vi "Pressure-Main-temp.vi"(8 "error in":errorcluster) -> (0 "error out":errorcluster)   [LabVIEW 2016]
doc: "Use this template to build a simple state machine design pattern. Each state executes code and determines which state to transition to."
uses:
  Controls/Pressure-Data.ctl
  Sensor-Class/Pressure-Transducer_class/Pressure-Transducer.lvclass
  Controls/Pressure-State.ctl
  Pressure Module.lvlib
panel:
  out "output array":u16[](array[numeric])
  out "Pressure":dbl[](array[numeric])
  out "Pressure 2":bool
  out "Status":string
  in  "Read Pressure":bool
  in  "Exit":bool
  # "P1"
  # "Flow 1"
  # "mA    Flow meter"
  # "Flow 2"
  # "mA  Flow meter"
  # "Top"
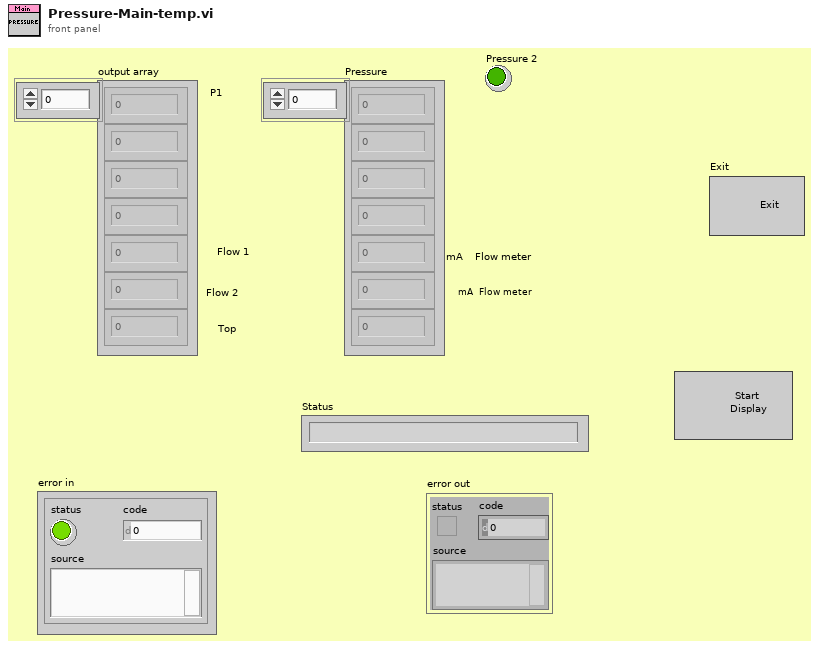
[diagram p1: front panel]
types:
  T1 = typedef "Pressure-State.ctl" = enum16{"Initialize", "Wait for Event", "Data: Pressure", "Data: Pressure-Sym", "Data: Display", "Data: Close", "Error", "Exit"}
  T2 = typedef "Pressure-Data.ctl" = cluster{"?":bool, "Status":string, "Pressure":dbl[], "Modbus-Instr":refnum<class "Pressure-Transducer.lvclass">}
  T3 = typedef "Pressure Module.lvlib/Request Events--cluster.ctl" = cluster{"Stop":refnum<user-event>, "Start Display Pressure":refnum<user-event>}
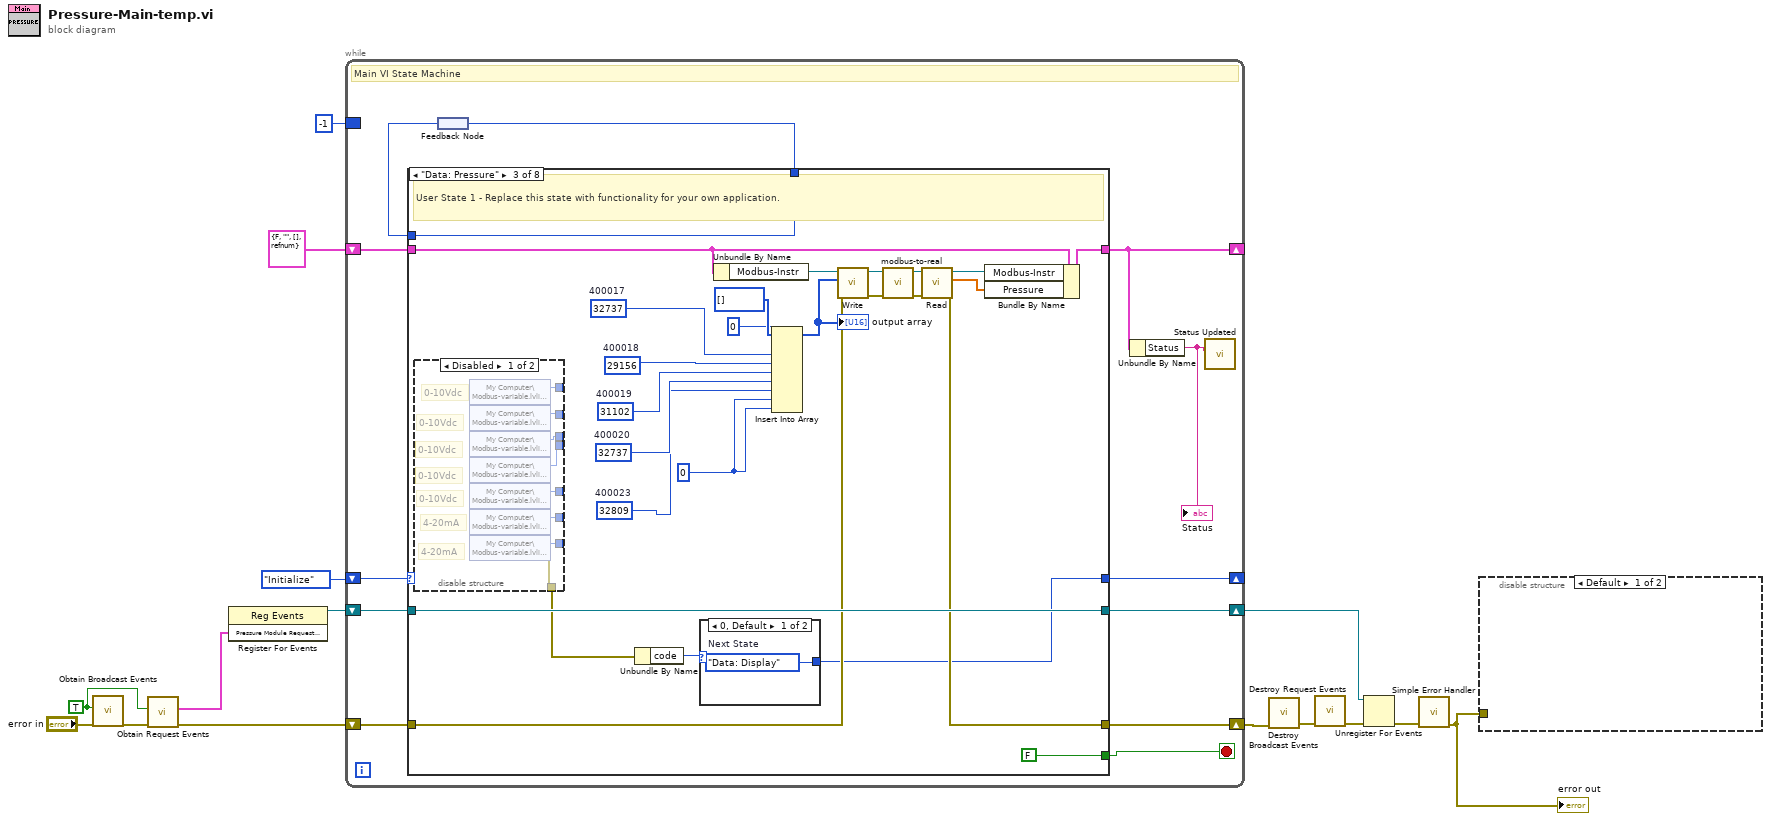
[diagram p0: block diagram]
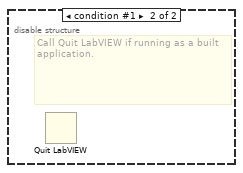
[diagram p2: hidden frame]
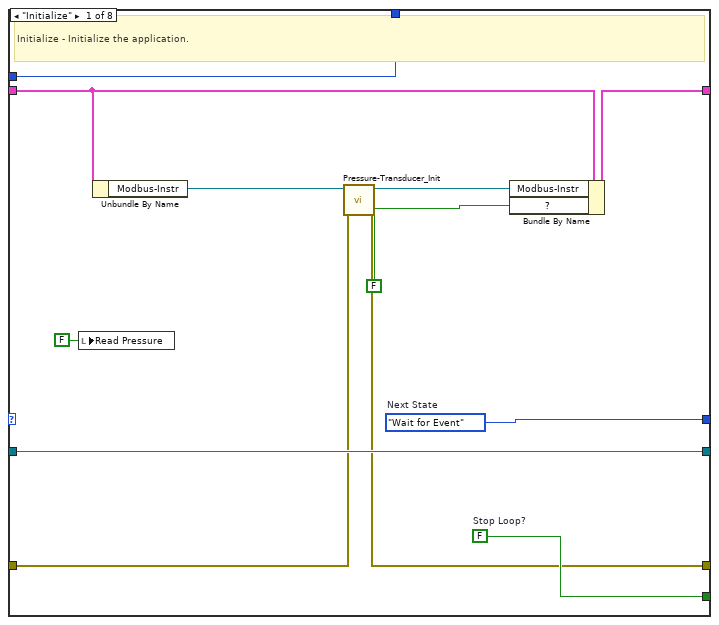
[diagram p3: hidden frame]
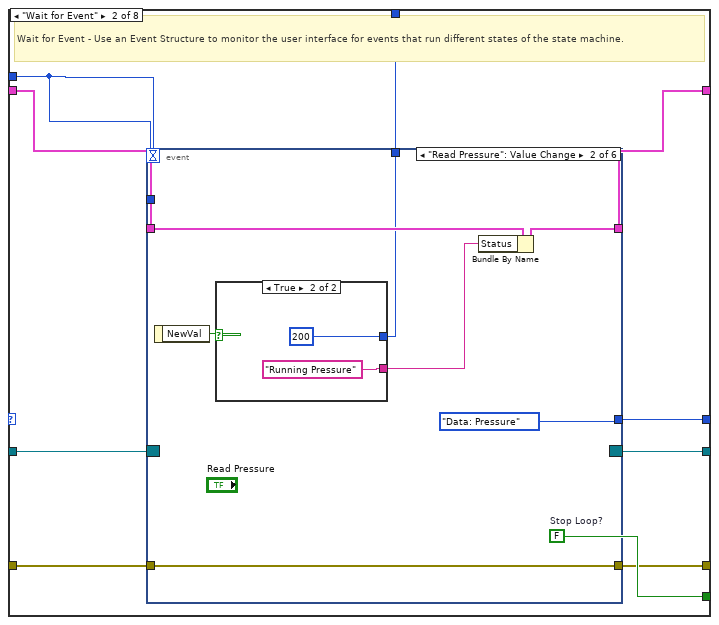
[diagram p4: hidden frame]
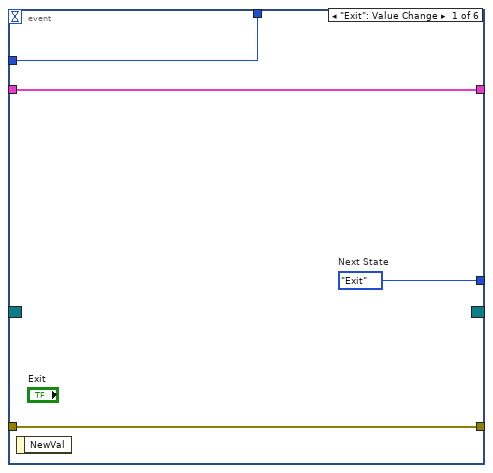
[diagram p5: hidden frame]
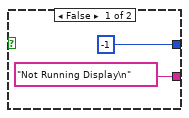
[diagram p6: hidden frame]
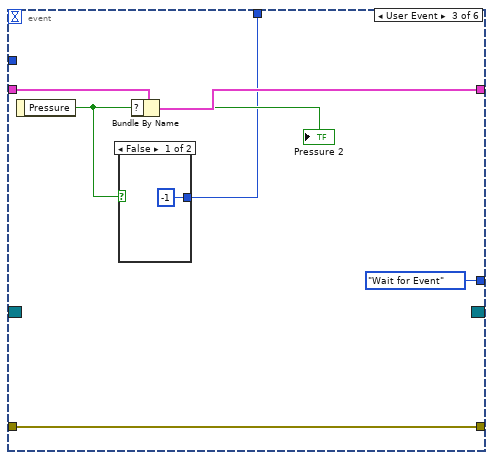
[diagram p7: hidden frame]
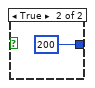
[diagram p8: hidden frame]
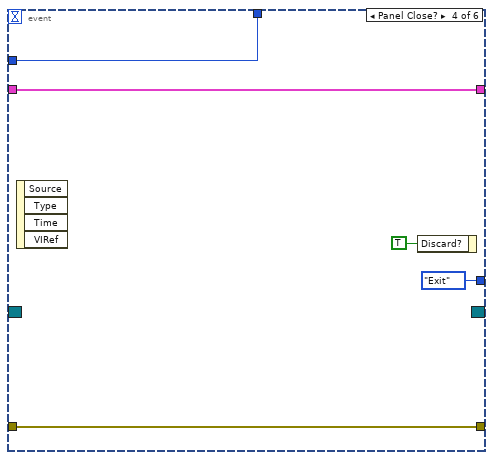
[diagram p9: hidden frame]
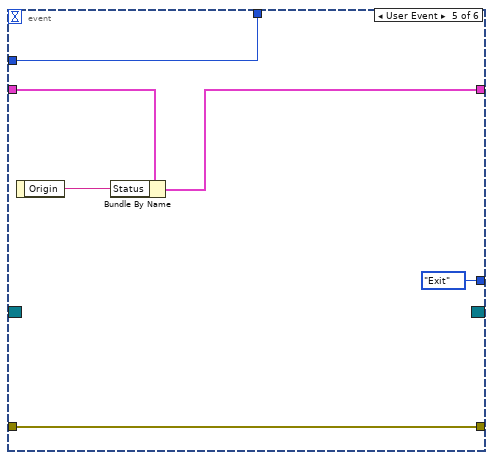
[diagram p10: hidden frame]
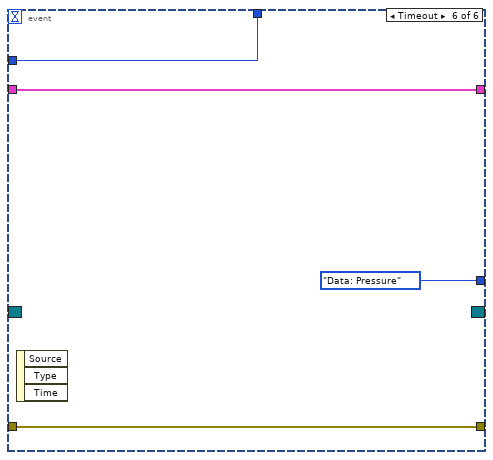
[diagram p11: hidden frame]
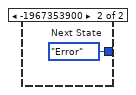
[diagram p13: hidden frame]
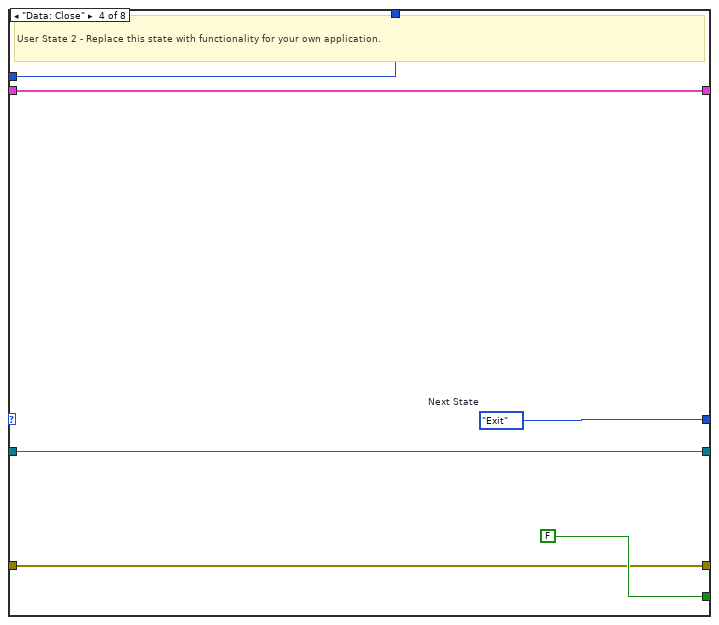
[diagram p14: hidden frame]
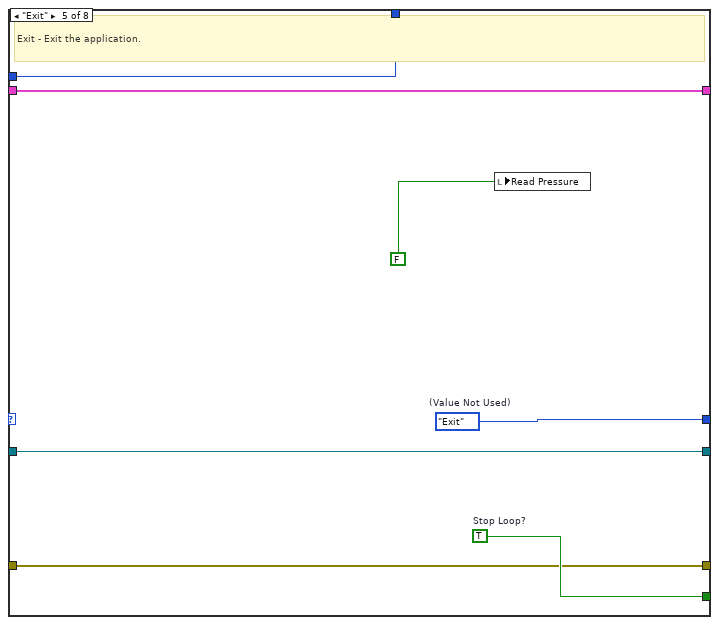
[diagram p15: hidden frame]
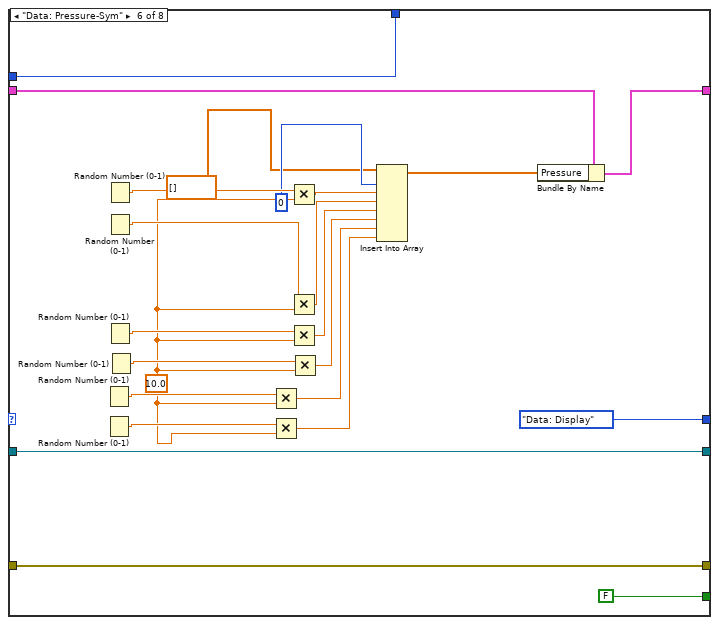
[diagram p16: hidden frame]
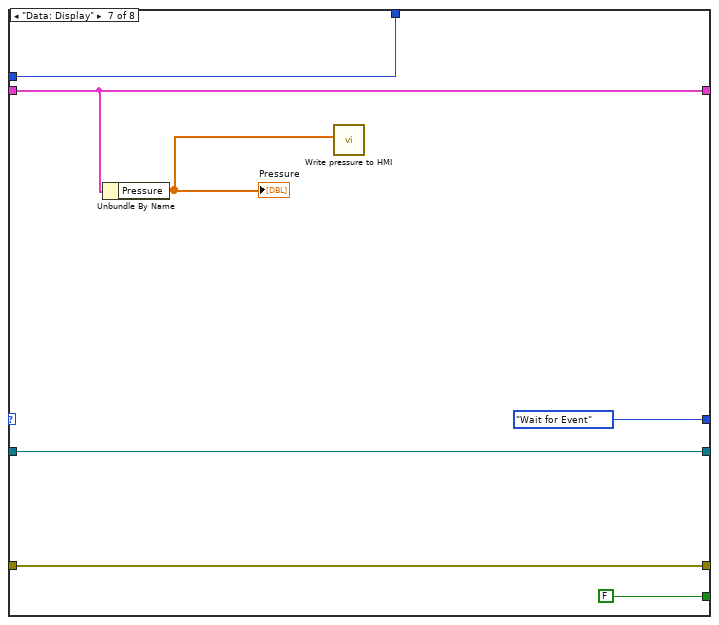
[diagram p17: hidden frame]
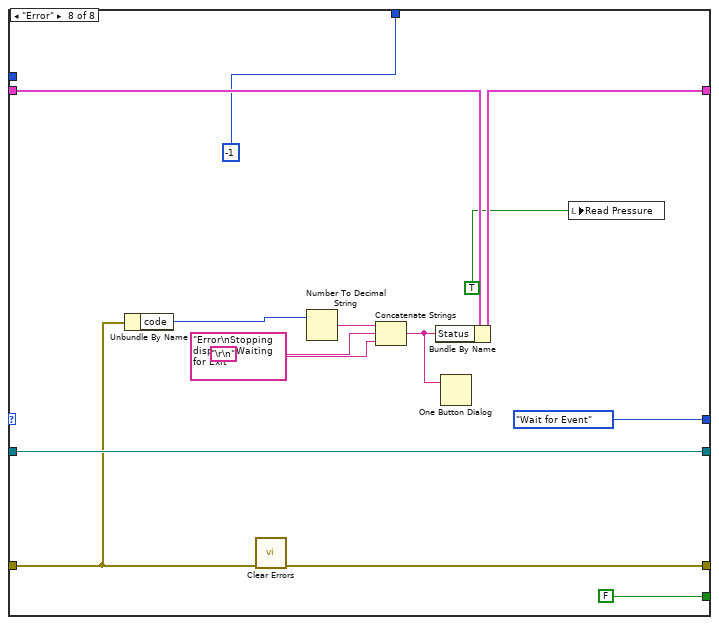
[diagram p18: hidden frame]
diagram:
  w10 = TRUE ("Create New?")
  n1 = call "Obtain Broadcast Events.vi"("error in (no error)"="error in", "Create New?"=w10) -> ("error out"=w13:errorcluster)  [unwired: 8 in, 1 out]
  n2 = call "Obtain Request Events.vi"("error in (no error)"=w13, "Create New?"=w10) -> ("error out"=w11:errorcluster, "Pressure Module Request Events"=w9:T3)  [unwired: 8 in]
  n3 = register-events(w9) -> (reference out=w8:refnum<event-registration>)  [unwired: 2 in, 1 out]
  n4 = while {
    shift-right: [w26] -> _
    shift-left: Pressure-State."Initialize" ("States") -> [w27]
    shift-right: [w19] -> _
    shift-left: T2 {"?"=FALSE, "Status"="", "Pressure"=[], "Modbus-Instr"=refnum} ("Data") -> [w25]
    shift-right: [w22] -> w5
    shift-left: w11 -> [w24]
    shift-right: [w21] -> w3
    shift-left: w8 -> [w20]
    border: -1 -> [_]
    stop <- w23 stop-if-true
    # "Main VI State Machine"
    n5 = feedback #1() -> (w17:i32)
    n6 = case shown="\"Data: Pressure\"" w27 {
      tunnel: [w39 w49 w95 w129 w136 Pressure-State."Data: Display" ("(Value Not Used)") Pressure-State."Wait for Event" ("(Value Not Used)") Pressure-State."Wait for Event" ("(Value Not Used)")] -> w26
      tunnel: [w38 w48 FALSE ("Stop Loop?") FALSE ("Stop Loop?") w134 FALSE ("Stop Loop?") FALSE ("Stop Loop?") FALSE ("Stop Loop?")] -> w23
      tunnel: w25 -> [w34 w47 w101 w127 w135 w143 w164 w178]
      tunnel: [w37 w46 w100 w127 w135 w142 w164 w177] -> w19
      tunnel: w24 -> [w31 w45 w103 w126 w133 w159 w166 w179]
      tunnel: [w30 w44 w102 w126 w133 w159 w166 w174] -> w22
      tunnel: [w35 w43 w112 w125 w132 w158 w165 w180] -> w21
      tunnel: w20 -> [w35 w42 w112 w125 w132 w158 w165 w180]
      tunnel: w17 -> [w29 w41 w94 w124 w131 w137 w160 _]
      tunnel: [w29 w40 w94 w124 w131 w137 w160 -1] -> w16
      frame "Initialize" {
        w38 = FALSE  # Stop Loop?
        w39 = Pressure-State."Wait for Event"  # Next State
        # "Initialize - Initialize the application."
        n7 = local write "Read Pressure"(FALSE ("Read Pressure")) -> ()
        n8 = Unbundle By Name(w34) -> ("Modbus-Instr"=w33:refnum<class "Pressure-Transducer.lvclass">)
        n9 = call "Pressure-Transducer_Init.vi"("error in (no error)"=w31, "object in"=w33) -> ("error out"=w30:errorcluster, "object out"=w32:refnum<class "Pressure-Transducer.lvclass">)  [unwired: 8 in]
        n10 = Bundle By Name(cluster=w34, "Modbus-Instr"=w32, "?"=FALSE ("Replace_Me_Boolean")) -> (w37:T2)
      }
      frame "Wait for Event" {
        w48 = FALSE  # Stop Loop?
        # "Wait for Event - Use an Event Structure to monitor the user interface for events that run different states of the state machine."
        n11 = event shown="[1] \"Read Pressure\": Value Change" {
          selector: w42 -> [_ _ _ _ _ _]
          dyn-events: [_ _ _ _ _ _] -> w43
          timeout: w41 -> [_ _ _ _ _ _]
          tunnel: [w53 Pressure-State."Data: Pressure" ("States") Pressure-State."Wait for Event" ("Initial State") Pressure-State."Exit" ("Initial State") Pressure-State."Exit" ("Initial State") Pressure-State."Data: Pressure" ("Initial State")] -> w49
          tunnel: w47 -> [w52 w60 w69 w77 w81 w86]
          tunnel: [w52 w59 w68 w77 w80 w86] -> w46
          tunnel: w45 -> [w51 w58 w70 w76 w83 w87]
          tunnel: [w51 w58 w70 w76 w83 w87] -> w44
          tunnel: w41 -> [w50 _ _ w73 w78 w84]
          tunnel: [w50 w55 w65 w73 w78 w84] -> w40
          event "Exit": Value Change {
            w53 = Pressure-State."Exit"  # Next State
            n12 = event-data() -> ()  [unwired: 1 in, 1 out]
          }
          event "Read Pressure": Value Change {
            n13 = event-data() -> ("NewVal"=w56:bool)  [unwired: 1 in]
            n14 = case shown="True" w56 {
              tunnel: [-1 200] -> w55
              tunnel: ["Not Running Display\n" ("Running User State 1") "Running Pressure" ("Running User State 1")] -> w54
              frame False {
              }
              frame True {
              }
            }
            n15 = Bundle By Name(cluster=w60, "Status"=w54) -> (w59:T2)
          }
          event User Event {
            n16 = event-data() -> ("Pressure"=w66:bool)  [unwired: 1 in]
            "Pressure 2" <- w66
            n17 = case shown="False" w66 {
              tunnel: [-1 200] -> w65
              frame False {
              }
              frame True {
              }
            }
            n18 = Bundle By Name(cluster=w69, "?"=w66) -> (w68:T2)
          }
          event Panel Close? {
            n19 = event-data() -> ()  [unwired: 1 in, 4 out]
            n20 = event-data("Discard?"=TRUE) -> ()  [unwired: 1 in, 1 out]
          }
          event User Event {
            n21 = event-data() -> ("Origin"=w79:string)  [unwired: 1 in]
            n22 = Bundle By Name(cluster=w81, "Status"=w79) -> (w80:T2)
          }
          event Timeout {
            n23 = event-data() -> ()  [unwired: 1 in, 3 out]
          }
        }
      }
      frame "Data: Pressure" {
        w90 = u16 32737  # 400020
        w91 = u16 31102  # 400019
        w88 = u16 0 ("400017")
        w89 = u16 32809  # 400023
        w92 = u16 29156  # 400018
        w93 = u16 32737  # 400017
        # "User State 1 - Replace this state with functionality for your own application."
        n24 = disable-structure shown="Disabled" {
          disable-tunnel: [w121 _] -> _
          disable-tunnel: [w120 _] -> _
          disable-tunnel: [w119 _] -> _
          disable-tunnel: [w118 _] -> _
          disable-tunnel: [w117 _] -> _
          disable-tunnel: [w116 _] -> _
          disable-tunnel: [w115 _] -> _
          disable-tunnel: [w114 _] -> w97
          frame Disabled {
            # "0-10Vdc"
            # "0-10Vdc"
            # "0-10Vdc"
            # "0-10Vdc"
            # "0-10Vdc"
            # "4-20mA"
            # "4-20mA"
            n25 = shared-variable "My Computer\\Modbus-variable.lvlib\\400017"() -> (w121:u16)  [unwired: 1 in, 1 out]
            n26 = shared-variable "My Computer\\Modbus-variable.lvlib\\400018"() -> (w120:u16)  [unwired: 1 in, 1 out]
            n27 = shared-variable "My Computer\\Modbus-variable.lvlib\\400019"() -> (w119:u16)  [unwired: 1 in, 1 out]
            n28 = shared-variable "My Computer\\Modbus-variable.lvlib\\400020"() -> (w118:u16)  [unwired: 1 in, 1 out]
            n29 = shared-variable "My Computer\\Modbus-variable.lvlib\\400021"() -> (w117:u16)  [unwired: 1 in, 1 out]
            n30 = shared-variable "My Computer\\Modbus-variable.lvlib\\400022"() -> (w116:u16)  [unwired: 1 in, 1 out]
            n31 = shared-variable "My Computer\\Modbus-variable.lvlib\\400023"() -> (w115:u16, error out=w114:errorcluster)  [unwired: 1 in]
          }
          frame Enabled {
          }
        }
        n32 = Unbundle By Name(w97) -> ("code"=w96:i32)
        n33 = case shown="0, Default" w96 {
          tunnel: [w122 w123] -> w95
          frame 0, Default {
            w122 = Pressure-State."Data: Display"  # Next State
          }
          frame -1967353900 {
            w123 = Pressure-State."Error"  # Next State
          }
        }
        n34 = Unbundle By Name(w101) -> ("Modbus-Instr"=w105:refnum<class "Pressure-Transducer.lvclass">)
        n35 = Insert Into Array(array=u16[] [], index=0, new element #1=w93, new element #2=w92, new element #3=w91, new element #4=w90, new element #5=w89, new element #6=w88, new element #7=w88) -> (w104:u16[])
        "output array" <- w104
        n36 = call-dynamic "Write.vi"("error in (no error)"=w103, "Modbus-Reg"=w104, "object in"=w105) -> ("error out"=w108:errorcluster, "object out"=w109:refnum<class "Pressure-Transducer.lvclass">)  [unwired: 7 in]
        n37 = call-dynamic "modbus-to-real.vi"("error in (no error)"=w108, "object in"=w109) -> ("error out"=w106:errorcluster, "object out"=w107:refnum<class "Pressure-Transducer.lvclass">)  [unwired: 8 in]
        n38 = call-dynamic "Read.vi"("error in (no error)"=w106, "object in"=w107) -> ("error out"=w102:errorcluster, "Data"=w98:dbl[], "object out"=w99:refnum<class "Pressure-Transducer.lvclass">)  [unwired: 7 in]
        n39 = Bundle By Name(cluster=w101, "Modbus-Instr"=w99, "Pressure"=w98) -> (w100:T2)
      }
      frame "Data: Close" {
        w129 = Pressure-State."Exit"  # Next State
        # "User State 2 - Replace this state with functionality for your own application."
      }
      frame "Exit" {
        w134 = TRUE  # Stop Loop?
        w136 = Pressure-State."Exit"  # (Value Not Used)
        # "Exit - Exit the application."
        n40 = local write "Read Pressure"(FALSE ("Read Pressure")) -> ()
      }
      frame "Data: Pressure-Sym" {
        w151 = 10.0 ("y")
        n41 = Random Number (0-1)() -> (number: 0 to 1=w153:dbl)
        n42 = Random Number (0-1)() -> (number: 0 to 1=w152:dbl)
        n43 = Random Number (0-1)() -> (number: 0 to 1=w157:dbl)
        n44 = Random Number (0-1)() -> (number: 0 to 1=w156:dbl)
        n45 = Random Number (0-1)() -> (number: 0 to 1=w155:dbl)
        n46 = Random Number (0-1)() -> (number: 0 to 1=w154:dbl)
        n47 = Multiply(x=w153, y=w151) -> (x*y=w145:dbl)
        n48 = Multiply(x=w152, y=w151) -> (x*y=w144:dbl)
        n49 = Multiply(x=w157, y=w151) -> (x*y=w149:dbl)
        n50 = Multiply(x=w156, y=w151) -> (x*y=w148:dbl)
        n51 = Multiply(x=w155, y=w151) -> (x*y=w147:dbl)
        n52 = Multiply(x=w154, y=w151) -> (x*y=w146:dbl)
        n53 = Insert Into Array(array=dbl[] [], index=0, new element #1=w149, new element #2=w148, new element #3=w147, new element #4=w146, new element #5=w145, new element #6=w144) -> (w141:dbl[])
        n54 = Bundle By Name(cluster=w143, "Pressure"=w141) -> (w142:T2)
      }
      frame "Data: Display" {
        n55 = Unbundle By Name(w164) -> ("Pressure"=w161:dbl[])
        "Pressure" <- w161
        n56 = call "Write pressure to HMI.vi"("Pressure"=w161) -> ()  [unwired: 10 in, 1 out]
      }
      frame "Error" {
        n57 = Unbundle By Name(w179) -> ("code"=w172:i32)
        n58 = call <vilib>:"Clear Errors.vi"("error in (no error)"=w179) -> ("error out"=w174:errorcluster)  [unwired: 5 in, 1 out]
        n59 = Number To Decimal String(number=w172) -> (decimal integer string=w171:string)  [unwired: 1 in]
        n60 = Concatenate Strings(w171, "\r\n", "Error\nStopping display\nWaiting for Exit" ("string")) -> (w168:string)
        n61 = Bundle By Name(cluster=w178, "Status"=w168) -> (w177:T2)
        n62 = One Button Dialog(message=w168) -> ()  [unwired: 1 in, 1 out]
        n63 = local write "Read Pressure"(TRUE ("Read Pressure")) -> ()
      }
    }
    n64 = feedback-in #1(w16) -> ()
    n65 = Unbundle By Name(w19) -> ("Status"=w18:string)
    "Status" <- w18
    n66 = call "Status Updated.vi"("Status"=w18) -> ()  [unwired: 10 in, 1 out]
  }
  n67 = call "Destroy Broadcast Events.vi"("error in (no error)"=w5) -> ("error out"=w7:errorcluster)  [unwired: 10 in]
  n68 = call "Destroy Request Events.vi"("error in (no error)"=w7) -> ("error out"=w6:errorcluster)  [unwired: 10 in]
  n69 = Unregister For Events(event registration refnum=w3, error in=w6) -> (error out=w4:errorcluster)
  n70 = call <vilib>:"Simple Error Handler.vi"("error in (no error)"=w4) -> ("error out"=w14:errorcluster)  [unwired: 4 in, 4 out]
  "error out" <- w14
  n71 = disable-structure shown="Default" {
    disable-tunnel: w14 -> [_ _]
    frame condition #0 (active) {
    }
    frame condition #1 {
      # "Call Quit LabVIEW if running as a built application."
      n72 = Quit LabVIEW() -> ()  [unwired: 1 in]
    }
  }
